vi "MCL Get Firmware Version.vi"(8 "error in (no error)":errorcluster, 9 "handle":i32, 10 "profile":i16, 11 "version":i16) -> (0 "error out":errorcluster, 1 "function return":i32, 2 "profile out":i16, 3 "version out":i16)   [LabVIEW 2014, in "Madlib.lvlib"]
doc: "MADLIB_API int MCL_GetFirmwareVersion(short *version, short *profile, int handle);"
uses:
  <userlib>/Lambda2/lib/Madlib/Madlib.lvlib
  <userlib>/Lambda2/lib/Madlib/Madlib.dll
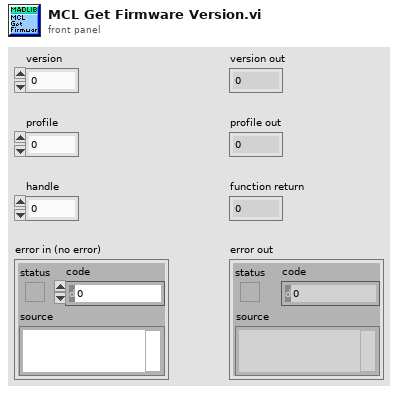
[diagram p1: front panel]
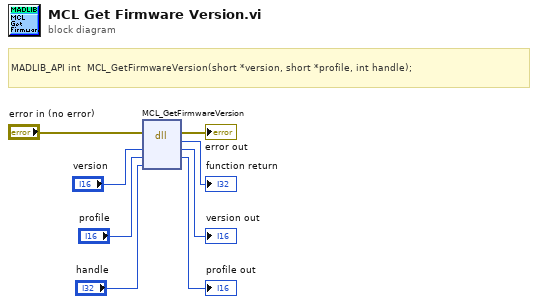
[diagram p0: block diagram]
diagram:
  # "MADLIB_API\tint \tMCL_GetFirmwareVersion(short *version, short *profile, int handle);"
  n1 = dll-call lib="C:/Program Files (x86)/National Instruments/LabVIEW 2014/user.lib/Lambda2/lib/Madlib/Madlib.*" fn="MCL_GetFirmwareVersion"(error in="error in (no error)", "version"="version", "profile"="profile", "handle"="handle") -> (error out=→"error out":errorcluster, →"function return":i32, "version"=→"version out":i16, "profile"=→"profile out":i16)  [unwired: 3 in, 1 out]
